vi "Set Parent.vi"(8 "error in (no error)":errorcluster, 11 "[MDI] Child in":refnum<class "[MDI] Child.lvclass">) -> (0 "error out":errorcluster, 3 "[MDI] Child out":refnum<class "[MDI] Child.lvclass">)   [LabVIEW 2020, in "[MDI] Child.lvlib" / "[MDI] Child.lvclass"]
uses:
  [MDI] Child.lvclass
  C:/Program Files (x86)/National Instruments/LabVIEW 2020/vi.lib/ActorFramework/Actor/Actor.lvclass
  <vilib>/ActorFramework/Actor/Actor.lvclass/Actor.ctl
  [MDI] Child.lvclass/[MDI] Child.ctl
  System.Windows.Forms
  [MDI] Parent/[MDI] Parent Messages/Add Child Msg/Add Child Msg.lvclass/Add Child Msg.ctl
  <vilib>/ActorFramework/Message Enqueuer/Message Enqueuer.lvclass/Message Enqueuer.ctl
  <vilib>/ActorFramework/Message Enqueuer/Enqueue.vi
  [MDI] Parent/[MDI] Parent Messages/Add Child Msg/Add Child Msg.lvclass
  C:/Program Files (x86)/National Instruments/LabVIEW 2020/vi.lib/ActorFramework/Message/Message.lvclass
  <vilib>/ActorFramework/Message Priority Queue/Priority Enqueue.vi
  user32.dll
  <vilib>/ActorFramework/Actor/Actor.lvclass
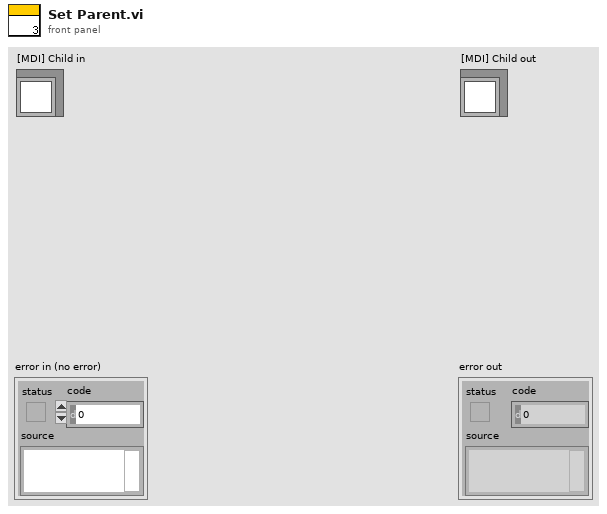
[diagram p1: front panel]
types:
  T1 = enum32{"Invalid", "Standard", "Closed", "Hidden", "Minimized", "Maximized"}
  T2 = typedef "LVRectTypeDef.ctl" = cluster{"Left":i16, "Top":i16, "Right":i16, "Bottom":i16}
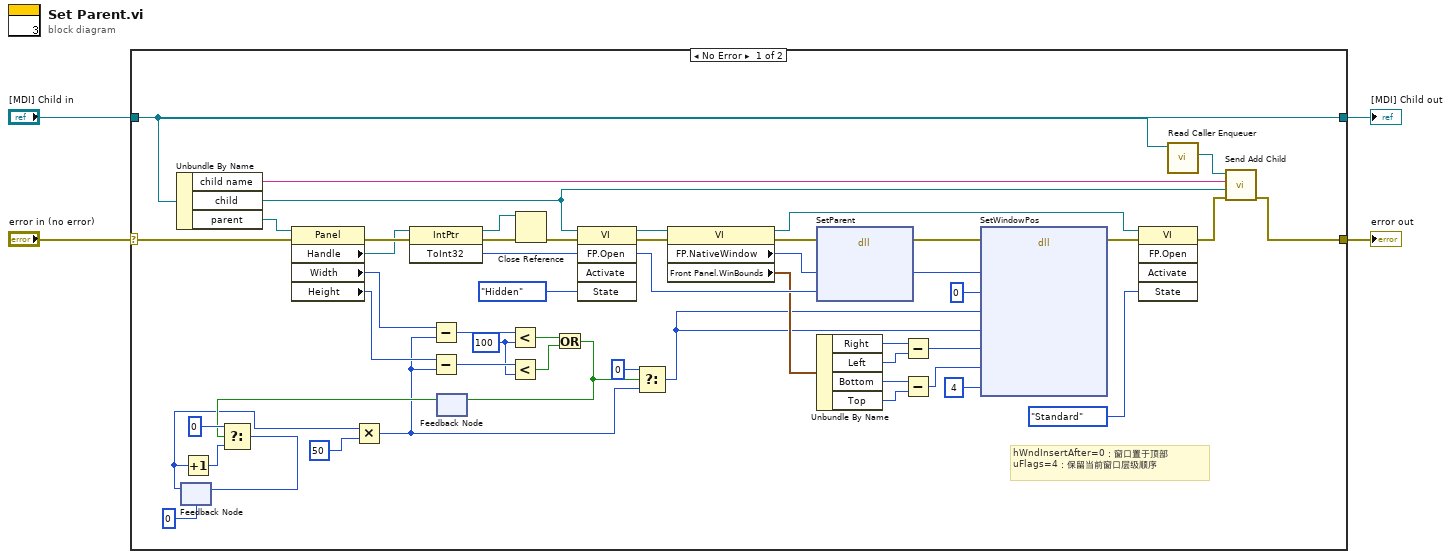
[diagram p0: block diagram]
diagram:
  n1 = case shown="No Error" "error in (no error)" {
    selector: "error in (no error)" -> [w49 w56]
    tunnel: [w7 w56] -> w3
    tunnel: [w11 w55] -> w1
    tunnel: "[MDI] Child in" -> [w11 w55]
    frame No Error {
      w34 = u32 100 ("y")
      # "hWndInsertAfter=0：窗口置于顶部\nuFlags=4：保留当前窗口层级顺序"
      n2 = Unbundle By Name(w11) -> ("child name"=w8:string, "child"=w5:refnum<vi>, "parent"=w53:refnum<k24>)
      n3 = feedback #1(u32 0 ("hWndInsertAfter")) -> (w29:u32)
      n4 = Increment(x=w29) -> (x+1=w30:u32)
      n5 = property class="Panel"(reference=w53, error in=w49) -> (error out=w54:errorcluster, "Handle"=w52:refnum<k24>, "Width"=w40:i32, "Height"=w39:i32)  [unwired: 1 out]
      n6 = Multiply(x=w29, y=u32 50) -> (x*y=w27:u32)
      n7 = invoke class="IntPtr" method="ToInt32"(reference=w52, error in=w54) -> (reference out=w47:refnum<k24>, error out=w48:errorcluster, "ToInt32"=w51:i32)  [unwired: 1 in]
      n8 = Subtract(x=w40, y=w27) -> (x-y=w36:u32)
      n9 = Subtract(x=w39, y=w27) -> (x-y=w35:u32)
      n10 = feedback #2() -> (w31:bool)  [unwired: 1 in]
      n11 = Select(t=u32 0, s=w31, f=w30) -> (s? t:f=w37:u32)
      n12 = feedback-in #1(w37) -> ()
      n13 = Less?(x=w36, y=w34) -> (x < y?=w33:bool)
      n14 = Less?(x=w35, y=w34) -> (x < y?=w32:bool)
      n15 = Close Reference(reference=w47, error in (no error)=w48) -> (error out=w45:errorcluster)
      n16 = Or(x=w33, y=w32) -> (x .or. y?=w28:bool)
      n17 = feedback-in #2(w28) -> ()
      n18 = invoke class="VI" method="FP.Open"(reference=w5, error in=w45, "State"=T1."Hidden") -> (error out=w44:errorcluster)  [unwired: 2 in, 4 out]
      n19 = Select(t=u32 0, s=w28, f=w27) -> (s? t:f=w26:u32)
      n20 = property class="VI"(reference=w5, error in=w44) -> (reference out=w23:refnum<vi>, error out=w46:errorcluster, "FP.NativeWindow"=w6:u64, "Front Panel.WinBounds"=w50:T2)
      n21 = dll-call lib="user32.dll" fn="SetParent"(error in=w46, "child"=w6, "newParent"=w51) -> (error out=w19:errorcluster, "child"=w21:u32)  [unwired: 4 in, 1 out]
      n22 = Unbundle By Name(w50) -> ("Right"=w17:i16, "Left"=w16:i16, "Bottom"=w15:i16, "Top"=w14:i16)
      n23 = Subtract(x=w17, y=w16) -> (x-y=w13:i16)
      n24 = Subtract(x=w15, y=w14) -> (x-y=w12:i16)
      n25 = dll-call lib="user32.dll" fn="SetWindowPos"(error in=w19, "hWnd"=w21, "hWndInsertAfter"=u32 0, "x"=w26, "y"=w26, "cx"=w13, "cy"=w12, "uFlags"=u32 4) -> (error out=w24:errorcluster)  [unwired: 10 in, 1 out]
      n26 = invoke class="VI" method="FP.Open"(reference=w23, error in=w24, "State"=T1."Standard") -> (error out=w10:errorcluster)  [unwired: 2 in, 4 out]
      n27 = call <vilib>:"Read Caller Enqueuer.vi"("Actor"=w11) -> ("Caller Enqueuer"=w9:refnum<class "Message Enqueuer.lvclass">)  [unwired: 10 in]
      n28 = call "Send Add Child.vi"("error in (no error)"=w10, "child"=w5, "child name"=w8, "Message Enqueuer"=w9) -> ("error out"=w7:errorcluster)  [unwired: 6 in, 1 out]
    }
    frame Error {
    }
  }
  "error out" <- w3
  "[MDI] Child out" <- w1
